vi "Meas Result Generate TWM Digitizer Correction - Generate CSV Matrix.vi"(4 "header":string, 5 "comment":string, 6 "amp [V]":dbl[](array[numeric]), 7 "CSV path":path, 8 "error in (no error)":errorcluster, 9 "uncertainty":dbl[][](array[numeric]), 10 "data":dbl[][](array[numeric]), 11 "f [Hz]":dbl[](array[numeric])) -> (0 "error out":errorcluster)   [LabVIEW 2020]
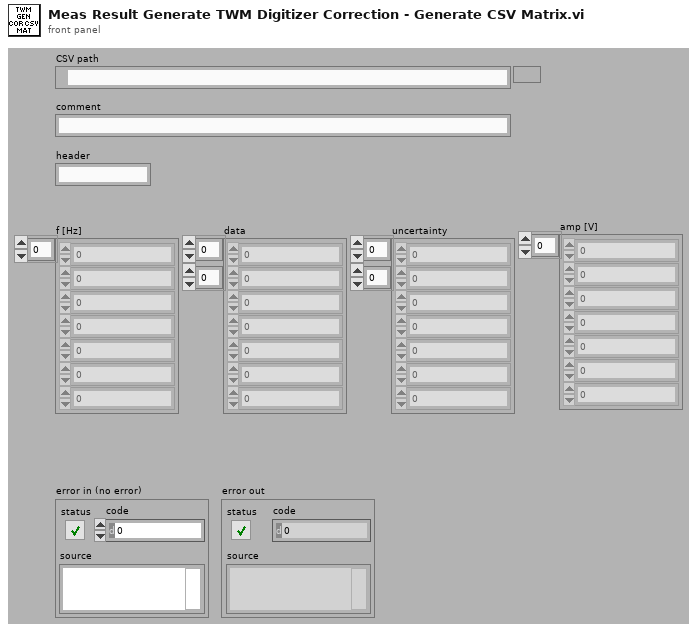
[diagram p1: front panel]
types:
  T1 = enum16{"open", "replace", "create", "open or create", "replace or create", "replace or create with confirmation"}
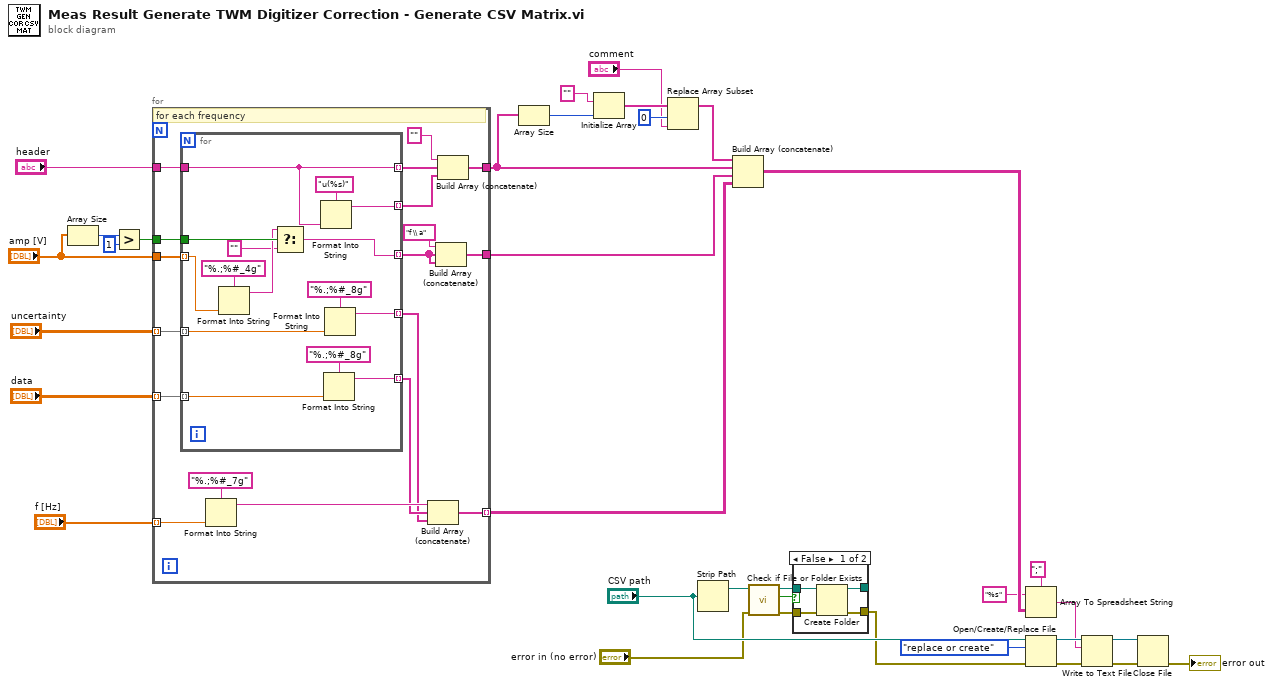
[diagram p0: block diagram]
diagram:
  n1 = Array Size(array="amp [V]") -> (size(s)=w3:i32)
  n2 = Greater?(x=w3, y=1) -> (0:w1:bool)
  n3 = for {
    tunnel: "f [Hz]" -> [w50] mode=indexing
    tunnel: "data" -> [w52] mode=indexing
    tunnel: "uncertainty" -> [w49] mode=indexing
    tunnel: [w45] -> w22 mode=indexing
    tunnel: [w42] -> w23
    tunnel: "header" -> [w41]
    tunnel: [w37] -> w24
    tunnel: "amp [V]" -> [w36]
    tunnel: w1 -> [w35]
    # "for each frequency"
    n4 = for {
      tunnel: w52 -> [w66] mode=indexing
      tunnel: w49 -> [w64] mode=indexing
      tunnel: [w63] -> w46 mode=indexing
      tunnel: [w62] -> w47 mode=indexing
      tunnel: [w53] -> w44 mode=indexing
      tunnel: w41 -> [w60]
      tunnel: [w60] -> w39 mode=indexing
      tunnel: [w59] -> w38 mode=indexing
      tunnel: w36 -> [w56] mode=indexing
      tunnel: w35 -> [w58]
      n5 = Format Into String(format string="%.;%#_4g", w56) -> (resulting string=w55:string)  [unwired: 2 in, 1 out]
      n6 = Select(t=w55, s=w58, f="") -> (s? t:f=w53:string)
      n7 = Format Into String(format string="u(%s)", w60) -> (resulting string=w59:string)  [unwired: 2 in, 1 out]
      n8 = Format Into String(format string="%.;%#_8g", w66) -> (resulting string=w62:string)  [unwired: 2 in, 1 out]
      n9 = Format Into String(format string="%.;%#_8g", w64) -> (resulting string=w63:string)  [unwired: 2 in, 1 out]
    }
    n10 = Format Into String(format string="%.;%#_7g", w50) -> (resulting string=w48:string)  [unwired: 2 in, 1 out]
    n11 = Build Array (concatenate)(w48, w47, w46) -> (w45:string[])
    n12 = Build Array (concatenate)("f \\ a", w44, w44) -> (w42:string[])
    n13 = Build Array (concatenate)("", w39, w38) -> (w37:string[])
  }
  n14 = Array Size(array=w24) -> (size(s)=w30:i32)
  n15 = Initialize Array("", w30) -> (w28:string[])
  n16 = Replace Array Subset(array=w28, new element="comment", index=0) -> (w25:string[])
  n17 = Strip Path(path="CSV path") -> (stripped path=w18:path)  [unwired: 1 out]
  n18 = Build Array (concatenate)(w25, w24, w23, w22) -> (w16:string[][])
  n19 = call <vilib>:"Check if File or Folder Exists.vi"("error in (no error)"="error in (no error)", "path"=w18) -> ("error out"=w19:errorcluster, "file or folder exists?"=w21:bool, "dup path"=w20:path)  [unwired: 7 in]
  n20 = case shown="False" w21 {
    tunnel: w20 -> [w71 w72]
    tunnel: [w70 w72] -> _
    tunnel: w19 -> [w69 w73]
    tunnel: [w68 w73] -> w12
    frame False {
      n21 = Create Folder(path (use dialog)=w71, error in=w69) -> (created path=w70:path, error out=w68:errorcluster)  [unwired: 1 in, 1 out]
    }
    frame True {
    }
  }
  n22 = Array To Spreadsheet String(delimiter (Tab)=";", array=w16, 3:"%s" ("format string")) -> (spreadsheet string=w8:string)
  n23 = Open/Create/Replace File(file path (use dialog)="CSV path", error in=w12, operation (0:open)=T1."replace or create") -> (refnum out=w9:refnum<file>, error out=w10:errorcluster)  [unwired: 3 in, 1 out]
  n24 = Write to Text File(file (use dialog)=w9, text=w8, error in=w10) -> (refnum out=w6:refnum<file>, error out=w7:errorcluster)  [unwired: 1 in, 1 out]
  n25 = Close File(refnum=w6, error in=w7) -> (error out=→"error out":errorcluster)  [unwired: 1 out]
